vi "DT_Triangle Manager_Find Ghost_by Point.vi"(10 "point":i32, 11 "Triangles":i32[][](array[numeric])) -> (0 "triangle 2":i32, 1 "point idx 1":i32, 2 "triangle 1":i32, 4 "point idx 2":i32)   [LabVIEW 2017, in "NI_AAL_Geometry.lvlib"]
uses:
  <vilib>/Analysis/NI_AAL_Geometry.lvlib
  <vilib>/Analysis/geometry.llb/DT_Triangle Manager_Get Global Point Index.vi
  <vilib>/Analysis/geometry.llb/DT_Triangle Manager_Get Adj_by Point.vi
  <vilib>/Analysis/geometry.llb/DT_Triangle Manager_Get Local Point Index.vi
  <vilib>/Analysis/geometry.llb/DT_Triangle Manager_Get Oppo Point_in Ghost.vi
  <vilib>/Analysis/geometry.llb/DT_Triangle Manager_Get Ghost Point.vi
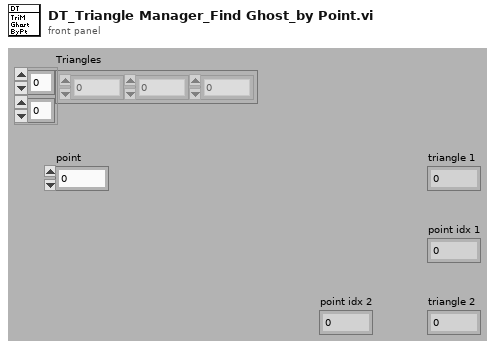
[diagram p1: front panel]
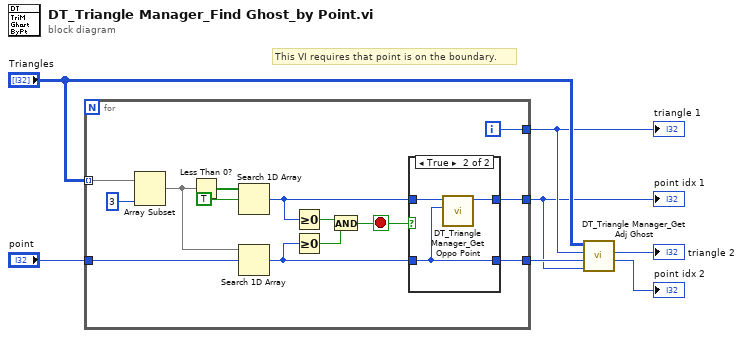
[diagram p0: block diagram]
diagram:
  # "This VI requires that point is on the boundary."
  n1 = for {
    tunnel: "Triangles" -> [w10] mode=indexing
    tunnel: "point" -> [w14]
    tunnel: [w18] -> w2
    tunnel: [w17] -> w5
    tunnel: [w16] -> w3
    i -> [w17]
    stop <- w19 stop-if-true
    n2 = Array Subset(array=w10, length=3) -> (w8:i32[])  [unwired: 1 in]
    n3 = Less Than 0?(x=w8) -> (x < 0?=w11:bool[])
    n4 = Search 1D Array(1D array=w11, element=TRUE) -> (index of element=w9:i32)  [unwired: 1 out]
    n5 = Search 1D Array(1D array=w8, element=w14) -> (index of element=w13:i32)  [unwired: 1 out]
    n6 = Greater Or Equal To 0?(x=w9) -> (x >= 0?=w21:bool)
    n7 = Greater Or Equal To 0?(x=w13) -> (x >= 0?=w20:bool)
    n8 = And(x=w21, y=w20) -> (x .and. y?=w19:bool)
    n9 = case shown="True" w19 {
      tunnel: w9 -> [_ w24]
      tunnel: w13 -> [_ w22]
      tunnel: [_ w23] -> w18
      tunnel: [_ w22] -> w16
      frame False {
      }
      frame True {
        n10 = call <vilib>:"DT_Triangle Manager_Get Oppo Point.vi"("point idx 2"=w22, "point idx 1"=w24) -> ("oppo point idx"=w23:i32)  [unwired: 9 out]
      }
    }
  }
  "triangle 1" <- w5
  "point idx 1" <- w2
  n11 = call <vilib>:"DT_Triangle Manager_Get Adj Ghost.vi"("cur point idx"=w2, "cur base point idx"=w3, "cur triangle"=w5, "Triangles In"="Triangles") -> ("next base point idx"=→"point idx 2":i32, "next triangle"=→"triangle 2":i32)  [unwired: 6 out]
